vi "To-simple-string.vi"(8 "error in (no error)":errorcluster, 11 "Home in":refnum<class "Home.lvclass">) -> (0 "error out":errorcluster, 2 "Action string":string, 3 "Home out":refnum<class "Home.lvclass">)   [LabVIEW 2013, in "PowderDeposition.lvlib" / "Home.lvclass"]
uses:
  Home.lvclass
  Home.lvclass/Home.ctl
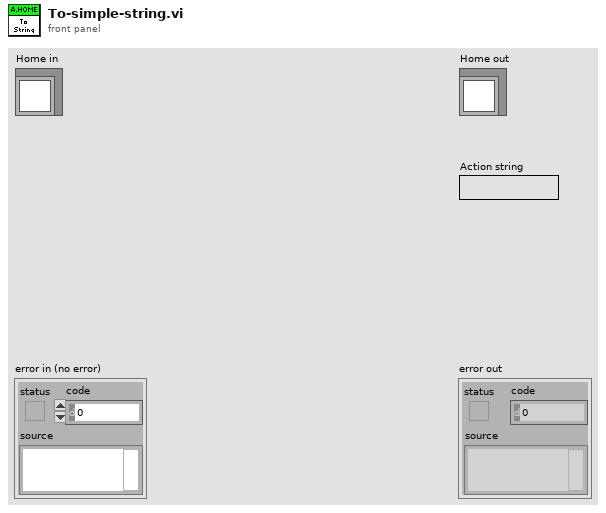
[diagram p1: front panel]
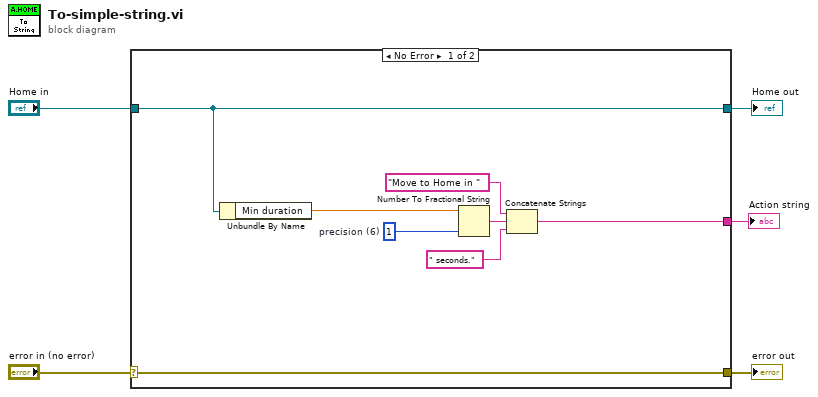
[diagram p0: block diagram]
diagram:
  n1 = case shown="No Error" "error in (no error)" {
    selector: "error in (no error)" -> [w13 w15]
    tunnel: [w13 w15] -> w4
    tunnel: [w8 w14] -> w2
    tunnel: "Home in" -> [w8 w14]
    tunnel: [w6 _] -> w1
    frame No Error {
      w9 = i16 1  # precision (6)
      n2 = Unbundle By Name(w8) -> ("Min duration"=w7:dbl)
      n3 = Number To Fractional String(number=w7, precision (6)=w9) -> (F-format string=w12:string)  [unwired: 2 in]
      n4 = Concatenate Strings("Move to Home in ", w12, " seconds.") -> (w6:string)
    }
    frame Error {
    }
  }
  "error out" <- w4
  "Home out" <- w2
  "Action string" <- w1
